vi "Modbus Master.vi"(7 "error in":errorcluster, 8 "Unit ID":u8=1, 9 "读取写入选择":string(combo), 10 "holding register values":u16[](array[numeric]) caption="写入保持寄存器的值", 11 "starting address":u16 caption="起始地址") -> (3 "register values":u16[](array[numeric]) caption="读取寄存器的值", 5 "error out":errorcluster)   [LabVIEW 2016, in "数据传输系统.lvlib"]
uses:
  <vilib>/NI/Modbus Library/API/Modbus API.lvclass/Modbus API.ctl
  <vilib>/NI/Modbus Library/Transmission Data Unit/Transmission Data Unit.lvclass/Transmission Data Unit.ctl
  <vilib>/NI/Modbus Library/API/Master/Set Unit ID.vi
  <vilib>/NI/Modbus Library/Transmission Data Unit/Write Unit ID.vi
  <vilib>/NI/Modbus Library/API/Read Transmission Data Unit.vi
  <vilib>/NI/Modbus Library/API/Write Transmission Data Unit.vi
  <vilib>/NI/Modbus Library/API/master/Modbus Master.lvclass
  D:/Program Files (x86)/National Instruments/LabVIEW 2016/vi.lib/NI/Modbus Library/API/Modbus API.lvclass
  <vilib>/NI/Modbus Library/API/Wrapper/Create TCP Master.vi
  <vilib>/NI/Modbus Library/API/Wrapper/API Main.lvlib
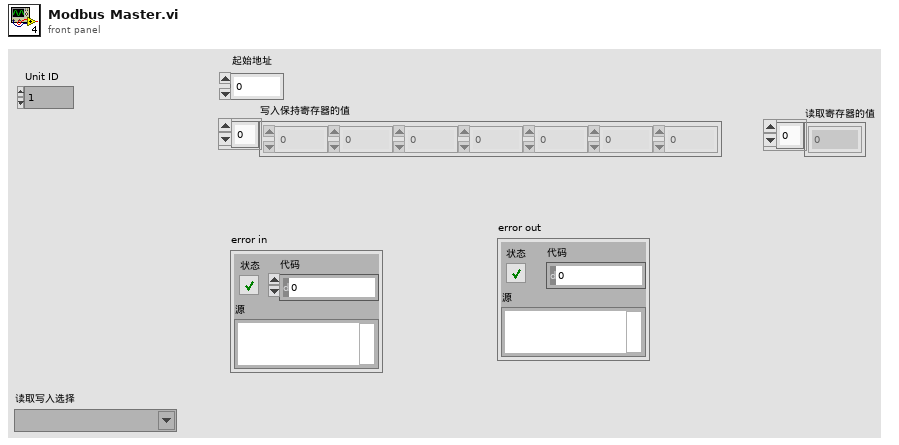
[diagram p1: front panel]
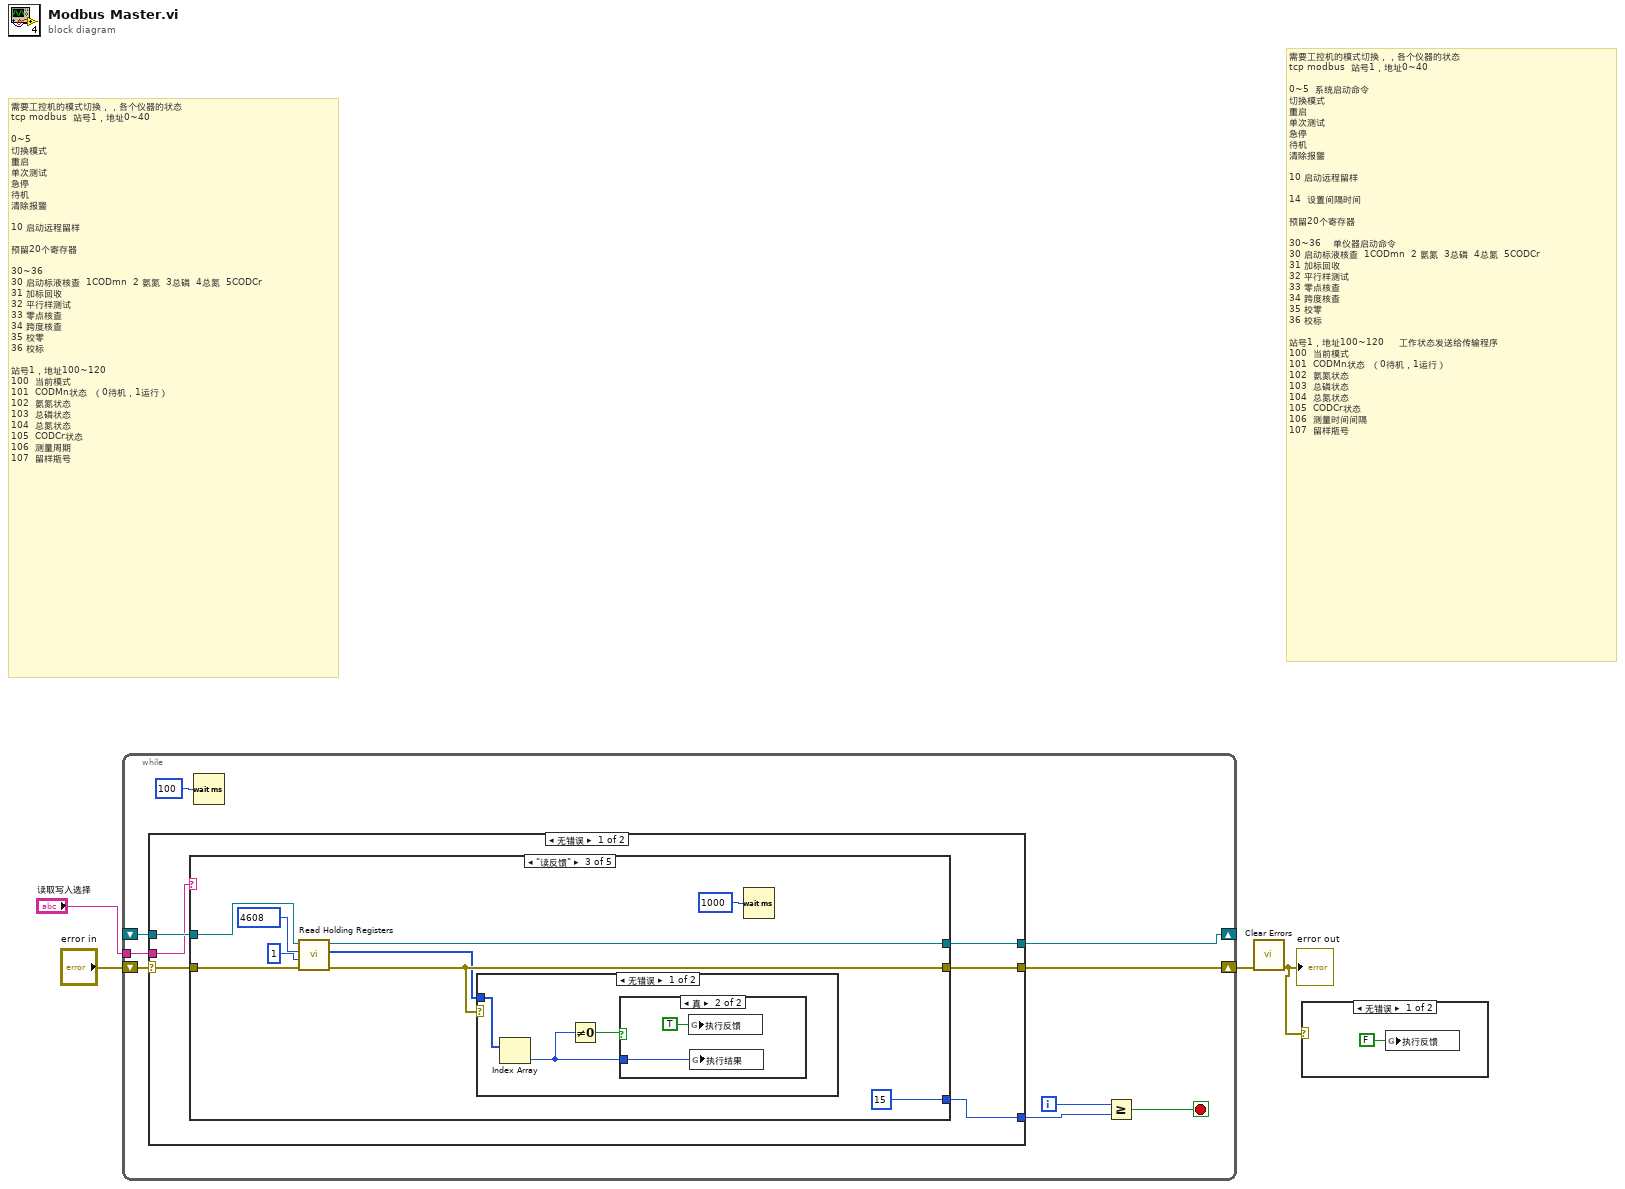
[diagram p0: block diagram]
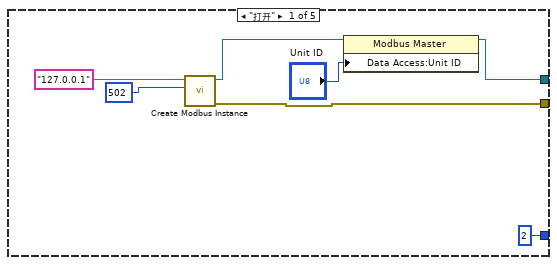
[diagram p3: hidden frame]
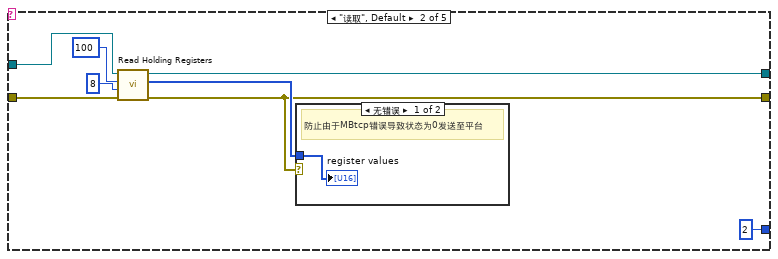
[diagram p4: hidden frame]
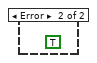
[diagram p7: hidden frame]
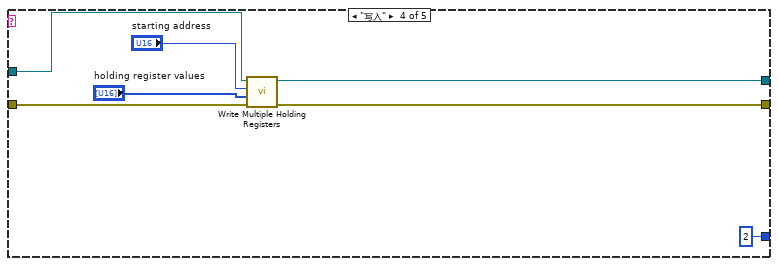
[diagram p8: hidden frame]
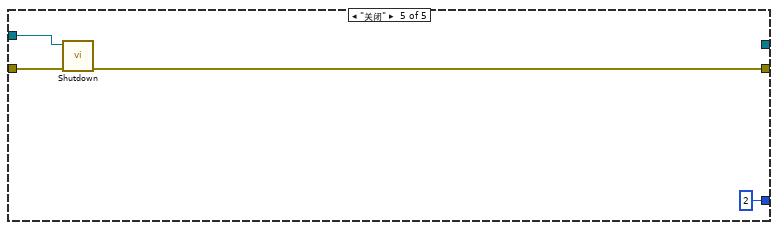
[diagram p9: hidden frame]
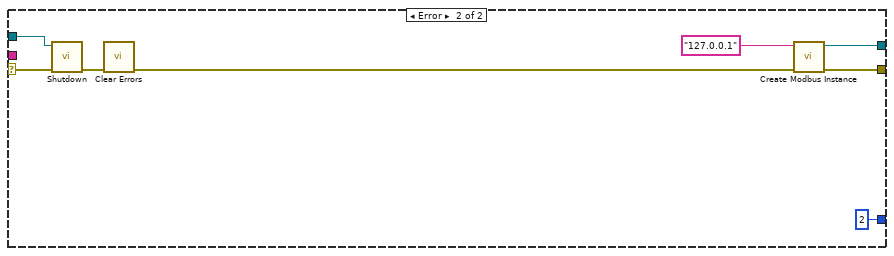
[diagram p10: hidden frame]
diagram:
  # "需要工控机的模式切换，，各个仪器的状态\ntcp modbus  站号1，地址0~40\n\n0~5  系统启动命令\n切换模式\n重启\n单次测试\n急停\n待机\n清除报警\n\n10 启动远程留样\n\n14  设置间隔时间\n\n预留20个寄存器\n\n30~36    单仪器启动命令\n30 启动标液核查  1CODmn  2 氨氮  3总磷  4总氮  5CODCr\n31 加标回收\n32 平行样测试\n33 零点核查\n34 跨度核查\n35 校零\n36 校标\n\n站号1，地址100~120     工作状态发送给传输程序\n100  当前模式\n101  CODMn状态  （0待机，1运行）\n102  氨氮状态\n103  总磷状态\n104  总氮状态\n105  CODCr状态\n106  测量时间间隔\n107  留样瓶号"
  # "需要工控机的模式切换，，各个仪器的状态\ntcp modbus  站号1，地址0~40\n\n0~5\n切换模式\n重启\n单次测试\n急停\n待机\n清除报警\n\n10 启动远程留样\n\n预留20个寄存器\n\n30~36\n30 启动标液核查  1CODmn  2 氨氮  3总磷  4总氮  5CODCr\n31 加标回收\n32 平行样测试\n33 零点核查\n34 跨度核查\n35 校零\n36 校标\n\n站号1，地址100~120\n100  当前模式\n101  CODMn状态  （0待机，1运行）\n102  氨氮状态\n103  总磷状态\n104  总氮状态\n105  CODCr状态\n106  测量周期\n107  留样瓶号"
  n1 = while {
    shift-right: [w7] -> w2
    shift-left: "error in" -> [w11]
    shift-right: [w12] -> _
    shift-left: _ -> [w13]
    tunnel: "读取写入选择" -> [w8]
    i -> [w9]
    stop <- w6 stop-if-true
    n2 = case shown="无错误" w11 {
      selector: w11 -> [w16 w62]
      tunnel: w13 -> [w19 w64]
      tunnel: [w18 w66] -> w12
      tunnel: [w17 w65] -> w7
      tunnel: w8 -> [w15 _]
      tunnel: [w14 2 ("y")] -> w5
      frame No Error {
        n3 = case shown="\"读反馈\"" w15 {
          tunnel: w19 -> [_ w34 w42 w56 w60]
          tunnel: [w23 w28 w40 w55 _] -> w18
          tunnel: [w22 w29 w39 w54 w58] -> w17
          tunnel: w16 -> [_ w33 w41 w53 w59]
          tunnel: [2 ("y") 2 ("y") 15 ("y") 2 ("y") 2 ("y")] -> w14
          frame "打开" {
            n4 = call-poly <vilib>:"Create Modbus Instance.vi"("port (502)"=u16 502, "address"="127.0.0.1") -> ("error out"=w22:errorcluster, "TCP master instance"=w26:refnum<class "Modbus Master.lvclass">)  [unwired: 8 in]
            n5 = property class="Modbus Master"(reference=w26, "Data Access:Unit ID"="Unit ID") -> (reference out=w23:refnum<class "Modbus Master.lvclass">)  [unwired: 1 in, 1 out]
          }
          frame "读取", Default {
            n6 = call-dynamic "Read Holding Registers.vi"("error in"=w33, "number of inputs"=u16 8 ("number of holding registers"), "starting address"=u16 100, "Modbus master in"=w34) -> ("error out"=w29:errorcluster, "register values"=w30:u16[], "Modbus master out"=w28:refnum<class "Modbus Master.lvclass">)  [unwired: 5 in]
            n7 = case shown="无错误" w29 {
              tunnel: w30 -> [w35 _]
              frame No Error {
                # "防止由于MBtcp错误导致状态为0发送至平台"
                "register values" <- w35
              }
              frame Error {
              }
            }
          }
          frame "读反馈" {
            n8 = call-dynamic "Read Holding Registers.vi"("error in"=w41, "number of inputs"=u16 1 ("number of holding registers"), "starting address"=u16 4608, "Modbus master in"=w42) -> ("error out"=w39:errorcluster, "register values"=w38:u16[], "Modbus master out"=w40:refnum<class "Modbus Master.lvclass">)  [unwired: 5 in]
            n9 = case shown="无错误" w39 {
              tunnel: w38 -> [w47 _]
              frame No Error {
                n10 = Index Array(array=w47) -> (element=w46:u16)  [unwired: 1 in]
                n11 = Not Equal To 0?(x=w46) -> (x != 0?=w45:bool)
                n12 = case shown="真" w45 {
                  tunnel: w46 -> [_ w48]
                  frame False {
                  }
                  frame True {
                    n13 = global write "全局 反控命令枚举.vi" "执行反馈"(TRUE ("执行反馈")) -> ()
                    n14 = global write "全局 反控命令枚举.vi" "执行结果"(w48) -> ()
                  }
                }
              }
              frame Error {
                (unwired) TRUE
              }
            }
            n15 = Wait (ms)(milliseconds to wait=u32 1000 ("等待时间（毫秒）")) -> ()  [unwired: 1 out]
          }
          frame "写入" {
            n16 = call-dynamic "Write Multiple Holding Registers.vi"("error in"=w53, "registers to write"="holding register values", "starting address"="starting address", "Modbus master in"=w56) -> ("error out"=w54:errorcluster, "Modbus master out"=w55:refnum<class "Modbus Master.lvclass">)  [unwired: 6 in]
          }
          frame "关闭" {
            n17 = call-dynamic "Shutdown.vi"("error in"=w59, "Modbus master in"=w60) -> ("error out"=w58:errorcluster)  [unwired: 9 in]
          }
        }
      }
      frame Error {
        n18 = call-dynamic "Shutdown.vi"("error in"=w62, "Modbus master in"=w64) -> ("error out"=w63:errorcluster)  [unwired: 9 in]
        n19 = call <vilib>:"Clear Errors.vi"("error in (no error)"=w63) -> ("error out"=w67:errorcluster)  [unwired: 5 in, 1 out]
        n20 = call-poly <vilib>:"Create Modbus Instance.vi"("error in"=w67, "address"="127.0.0.1") -> ("error out"=w65:errorcluster, "TCP master instance"=w66:refnum<class "Modbus Master.lvclass">)  [unwired: 8 in]
      }
    }
    n21 = Wait (ms)(milliseconds to wait=u32 100 ("等待时间（毫秒）")) -> ()  [unwired: 1 out]
    n22 = Greater Or Equal?(x=w9, y=w5) -> (x >= y?=w6:bool)
  }
  n23 = call <vilib>:"Clear Errors.vi"("error in (no error)"=w2) -> ("error out"=w1:errorcluster)  [unwired: 5 in, 1 out]
  "error out" <- w1
  n24 = case shown="无错误" w1 {
    frame No Error {
      n25 = global write "全局 反控命令枚举.vi" "执行反馈"(FALSE ("执行反馈")) -> ()
    }
    frame Error {
    }
  }
